vi "DQ_Conjugate.vi"(1 "DQ2":cluster{"q":T1, "qe":T1}) -> (0 "Conjugate":cluster{"q":T1, "qe":T1})   [LabVIEW 2014]
doc: "产生四元数的共轭四元数"
uses:
  <vilib>/robotics/Kinematics/Quaternion.ctl
  <vilib>/robotics/Kinematics/NI_Kinematics.lvlib
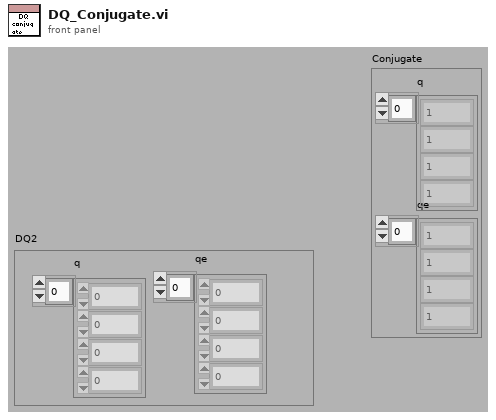
[diagram p1: front panel]
types:
  T1 = typedef "NI_Kinematics.lvlib/Quaternion.ctl" = dbl[]
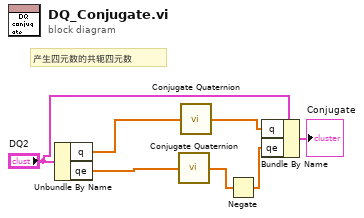
[diagram p0: block diagram]
diagram:
  # "产生四元数的共轭四元数"
  n1 = Unbundle By Name("DQ2") -> ("q"=w6:T1, "qe"=w5:T1)
  n2 = call <vilib>:"Conjugate Quaternion.vi"("quaternion"=w5) -> ("conjugate"=w2:T1)
  n3 = call <vilib>:"Conjugate Quaternion.vi"("quaternion"=w6) -> ("conjugate"=w3:T1)
  n4 = Negate(x=w2) -> (-x=w1:T1)
  n5 = Bundle By Name(cluster="DQ2", "q"=w3, "qe"=w1) -> (→"Conjugate":cluster{"q":T1, "qe":T1})
